vi "cathodicFitTest.vi"() -> ()   [LabVIEW 2018]
uses:
  <vilib>/Utility/file.llb/Read Delimited Spreadsheet (DBL).vi
panel:
  out "fitConstants":dbl[](array[numeric])=[-0.4886252489079526, -0.041148610014685456]
  out "Array 2":dbl[](array[numeric])=[-0.286073, -0.36550535885320207]
  out "Array":dbl[](array[numeric])=[0.007281221461747875, 0.050183]
  out "corrCoeffVals":dbl[](array[numeric])=[nan, -0.9999999854897975, -0.9999989757932266, -0.9999931848952519, -0.9999856896532151, -0.9999860250090599, -0.9999637800289322, -0.9999644118485376, -0.999964942406983, -0.9999613481711687, -0.9999316333038044, -0.9999322944047723, -0.9999328696887111, -0.9999333743940425, -0.9999338204636762, -0.9999342173736078, -0.9999345727025364, -0.9999348925701779, -0.9999351819817387, -0.9999354450452024, -0.9999356851571781, 0.9999244057562761, 0.9998864677799435, 0.9998867995146092, 0.9998871065211875, 0.9998637876975295, 0.999763096945273, 0.9997636184039532, 0.999686087744513, 0.9996866956204068, 0.9996738333542307, 0.999548708251031, 0.9995438504085573, 0.9994441087829002, 0.9994129500518916, 0.999252267957993, 0.9992532442311977, 0.9991015406036009, 0.998931131055494, 0.9987186624806976, 0.9986201773705358, 0.9983163038792315, 0.9982110360592806, 0.9977027898521647, 0.9976048241443399, 0.9976068831687861, 0.9975748525102933, 0.9972726871270071, 0.9970432759444724, 0.997045439656857, 0.9970475212425098, 0.9968871800862679, 0.9966761545684867, 0.9966782507846038, 0.9962447080502259, 0.9962469137507166, 0.9960013895295876, 0.9955800868241822, 0.9952113737706112, 0.994971805263109, 0.9949436775443121, 0.9944287307646397, 0.9943289970691769, 0.9943315581408776, 0.9934163617136997, 0.9934191562963511, 0.9929350972397707, 0.9929379240121593, 0.9906827961841149, 0.9906862995776826, 0.9905793873858413, 0.9901282346317134, 0.9901316512689583, 0.988218807777571, 0.988222657384164, 0.987579045404995, 0.9873577920316247, 0.9845720093200628, 0.9838996527549713, 0.9815319874531447, 0.9815370927365834, 0.981067272838562, 0.9787389103943759, 0.9784632707995644, 0.9769895185248851, 0.9718633867432568, 0.9673537842474299, 0.967361180380475, 0.9673684140630285, 0.9632586334805677, 0.9571459046270959, 0.9525515935812403, 0.9496770949348121, 0.9453242203109834, 0.9254767471982777, 0.9254894457474564, 0.892096111414348, 0.0, 0.0, 0.0, 0.0, 0.0, 0.0, 0.0, 0.0, 0.0, 0.0, 0.0, 0.0, 0.0, 0.0, 0.0, 0.0, 0.0, 0.0, 0.0, 0.0, 0.0, 0.0, 0.0, 0.0, 0.0, 0.0, 0.0, 0.0, 0.0, 0.0, 0.0, 0.0, 0.0, 0.0, 0.0, 0.0, 0.0, 0.0, 0.0, 0.0, 0.0, 0.0, 0.0, 0.0, 0.0, 0.0, 0.0, 0.0, 0.0, 0.0, 0.0, 0.0, 0.0, 0.0, 0.0, 0.0, 0.0, 0.0, 0.0, 0.0, 0.0, 0.0, 0.0, 0.0, 0.0, 0.0, 0.0, 0.0, 0.0, 0.0, 0.0, 0.0, 0.0, 0.0, 0.0, 0.0, 0.0, 0.0, 0.0, 0.0, 0.0, 0.0, 0.0, 0.0, 0.0, 0.0, 0.0, 0.0, 0.0, 0.0, 0.0, 0.0, 0.0, 0.0, 0.0, 0.0, 0.0, 0.0, 0.0, 0.0, 0.0, 0.0, 0.0]
  out "return type":dbl
  out "cathodicElements":i32=89
  out "eCorr":dbl=-0.286073
  in  "corrCoeff":dbl=0.96 step=0.01 format="%#_13g"
  in  "yData Filename":string="yData2"
  in  "xData Filename":string="xData2"
  out "error out":errorcluster
  out "MEASUREMENT":cluster{"XCoords":dbl[], "YCoords":dbl[]}[](graph)=[{"XCoords"=array[332 elements], "YCoords"=array[332 elements]}, {"XCoords"=[0.007281221461747875, 0.050183], "YCoords"=[-0.286073, -0.36550535885320207]}]
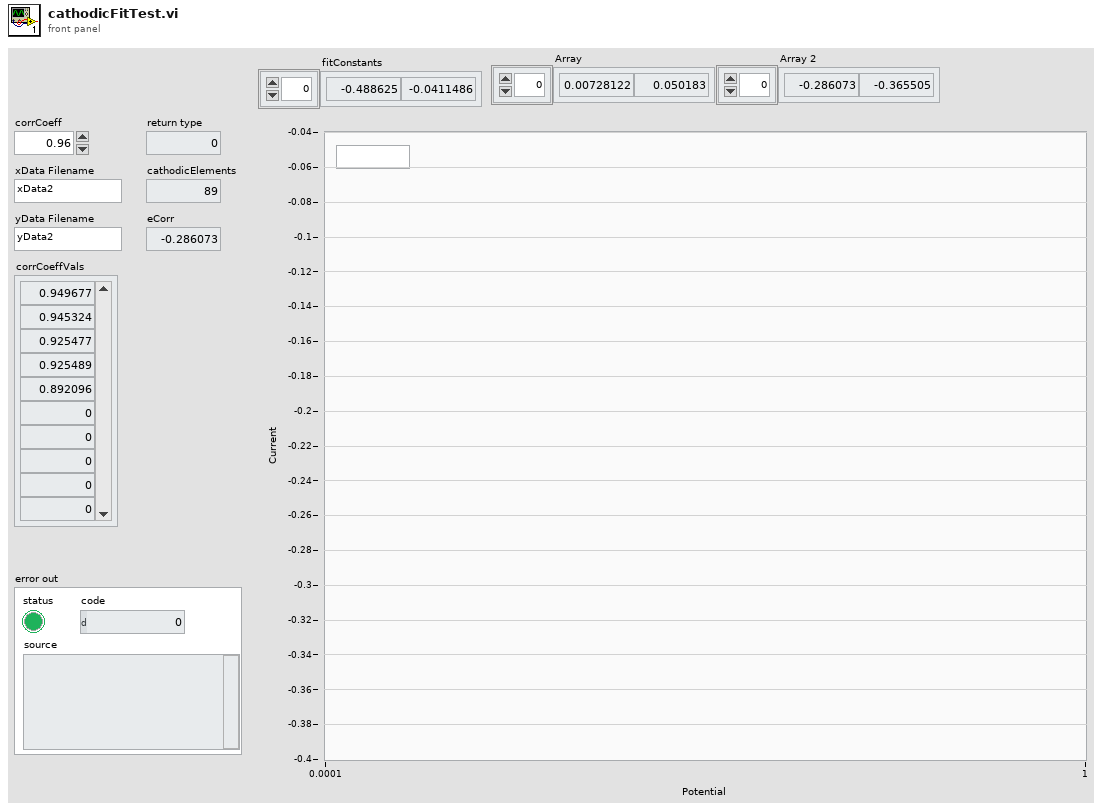
[diagram p1: front panel]
types:
  T1 = cluster{"CathodicFit":cluster{"XCoords":dbl[], "YCoords":dbl[]}}
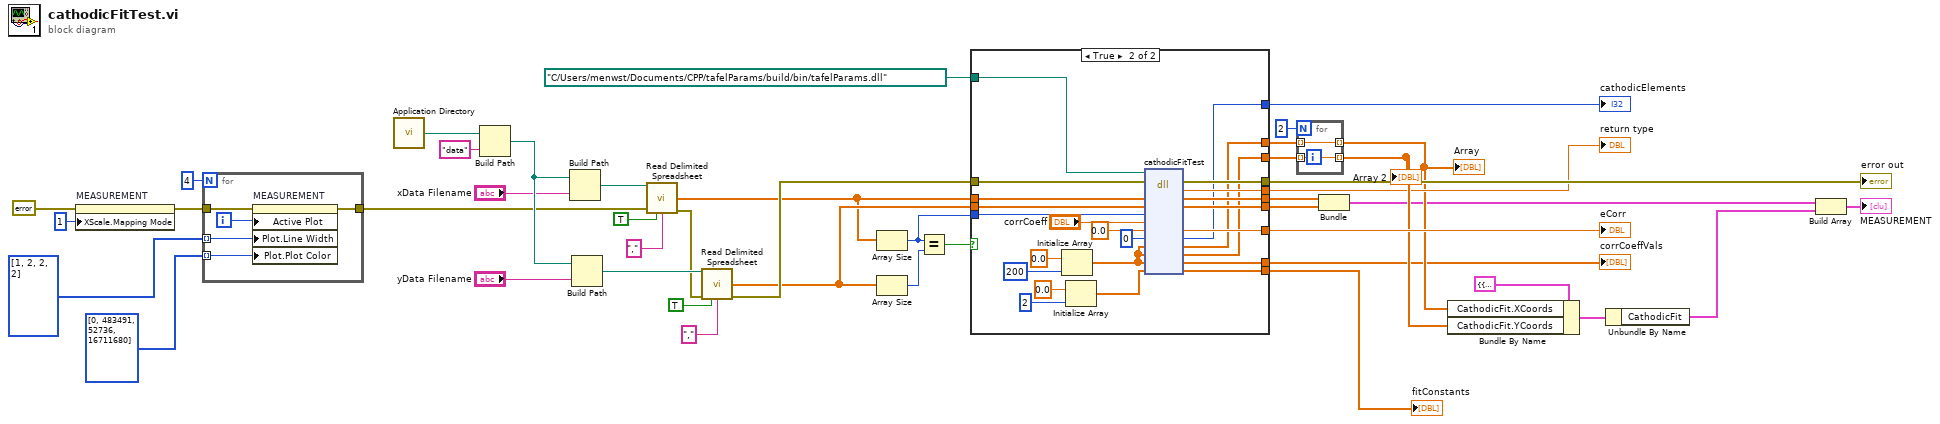
[diagram p0: block diagram]
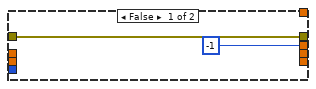
[diagram p2: hidden frame]
diagram:
  n1 = property on="MEASUREMENT" class="XYGraph (strict)"(error in=errorcluster {"status"=FALSE, "code"=0, "source"=""} ("error out"), "XScale.Mapping Mode"=u8 1 ("X Scale.Mapping Mode")) -> (error out=w21:errorcluster)  [unwired: 1 in, 1 out]
  n2 = for {
    N: 4 -> [_]
    tunnel: w21 -> [w48]
    tunnel: [w47] -> w20
    tunnel: u32[] [0, 483491, 52736, 16711680] -> [w46] mode=indexing
    tunnel: i32[] [1, 2, 2, 2] -> [w45] mode=indexing
    i -> [w49]
    n3 = property on="MEASUREMENT" class="XYGraph (strict)"(error in=w48, "Active Plot"=w49, "Plot.Line Width"=w45, "Plot.Plot Color"=w46) -> (error out=w47:errorcluster)  [unwired: 1 in, 1 out]
  }
  n4 = call <vilib>:"Application Directory.vi"() -> ("Application Directory"=w40:path)
  n5 = Build Path(base path=w40, name or relative path="data") -> (appended path=w38:path)
  n6 = Build Path(base path=w38, name or relative path="xData Filename") -> (appended path=w35:path)
  n7 = Build Path(base path=w38, name or relative path="yData Filename") -> (appended path=w34:path)
  n8 = call-poly <vilib>:"Read Delimited Spreadsheet.vi"("file path (dialog if empty)"=w35, "error in (no error)"=w20, "transpose? (F)"=TRUE, "delimiter (\\t)"="," ("delimiter (\\t)")) -> ("first row"=w15:dbl[], "error out"=w32:errorcluster)  [unwired: 6 in, 4 out]
  n9 = call-poly <vilib>:"Read Delimited Spreadsheet.vi"("file path (dialog if empty)"=w34, "error in (no error)"=w32, "transpose? (F)"=TRUE, "delimiter (\\t)"="," ("delimiter (\\t)")) -> ("first row"=w16:dbl[], "error out"=w31:errorcluster)  [unwired: 6 in, 4 out]
  n10 = Array Size(array=w15) -> (size(s)=w25:i32)
  n11 = Array Size(array=w16) -> (size(s)=w30:i32)
  n12 = Equal?(x=w25, y=w30) -> (x = y?=w29:bool)
  n13 = case shown="True" w29 {
    tunnel: [w50 w75] -> w14
    tunnel: [-1 ("return type") w74] -> w9
    tunnel: w16 -> [_ w68]
    tunnel: w15 -> [_ w69]
    tunnel: w31 -> [w50 w73]
    tunnel: path "C:/Users/menwst/Documents/CPP/tafelParams/build/bin/tafelParams.dll" ("path in") -> [_ w72]
    tunnel: [_ w66] -> w4
    tunnel: [_ w65] -> w17
    tunnel: w25 -> [_ w67]
    tunnel: [_ w60] -> w13
    tunnel: [_ w59] -> w3
    tunnel: [_ w58] -> w12
    tunnel: [_ w57] -> w11
    tunnel: [_ w56] -> w7
    tunnel: [_ w52] -> w1
    frame False {
    }
    frame True {
      n14 = Initialize Array(0.0 ("element"), 200 ("xnumRows")) -> (w61:dbl[])
      n15 = Initialize Array(0.0 ("element"), 2 ("xnumRows")) -> (w53:dbl[])
      n16 = dll-call lib="C:/Users/menwst/Documents/CPP/tafelParams/build/bin/tafelParams.dll" fn="cathodicFitTest"(path in=w72, error in=w73, "xdata"=w69, "ydata"=w68, "numRows"=w67, "cathodicCorrCoeff"="corrCoeff", "eCorr"=0.0 ("element"), "cathodicElements"=0 ("intersects"), "xCathodicFit"=w61, "yCathodicFit"=w61, "corrCoeffVals"=w61, "fitConstants"=w53) -> (error out=w75:errorcluster, "return type"=w74:dbl, "xdata"=w66:dbl[], "ydata"=w65:dbl[], "eCorr"=w60:dbl, "cathodicElements"=w59:i32, "xCathodicFit"=w58:dbl[], "yCathodicFit"=w57:dbl[], "corrCoeffVals"=w56:dbl[], "fitConstants"=w52:dbl[])  [unwired: 3 in, 1 out]
    }
  }
  "error out" <- w14
  "eCorr" <- w13
  "cathodicElements" <- w3
  "return type" <- w9
  "corrCoeffVals" <- w7
  "fitConstants" <- w1
  n17 = for {
    N: 2 -> [_]
    tunnel: w12 -> [w77] mode=indexing
    tunnel: w11 -> [w76] mode=indexing
    tunnel: [w77] -> w8 mode=indexing
    tunnel: [w76] -> w10 mode=indexing
  }
  "Array" <- w8
  "Array 2" <- w10
  n18 = Bundle("xdata"=w4, "ydata"=w17) -> (w6:cluster{"xdata":dbl[], "ydata":dbl[]})  [unwired: 1 in]
  n19 = Bundle By Name(cluster=T1 {"CathodicFit"={"XCoords"=[], "YCoords"=[]}} ("Fit Coords"), "CathodicFit.XCoords"=w8, "CathodicFit.YCoords"=w10) -> (w27:T1)
  n20 = Unbundle By Name(w27) -> ("CathodicFit"=w26:cluster{"XCoords":dbl[], "YCoords":dbl[]})
  n21 = Build Array(w6, w26) -> (→"MEASUREMENT":cluster{"XCoords":dbl[], "YCoords":dbl[]}[])
